vi "Write Data Type.vi"(8 "error in (no error)":errorcluster, 10 "Data Type":T1, 11 "OnChange_Boolean in":refnum<class "OnChangeNotifier_I8.lvclass">) -> (0 "error out":errorcluster, 3 "OnChange_Boolean out":refnum<class "OnChangeNotifier_I8.lvclass">)   [LabVIEW 2021, in "OnChangeNotifier_I8.lvclass"]
uses:
  OnChangeNotifier_I8.lvclass
  Support/Class Type.ctl
  OnChangeNotifier_I8.lvclass/OnChangeNotifier_I8.ctl
  <vilib>/TSA/Abstract Data Classes/Abs_Types/I8 Integer/Abs_I8 Integer.lvclass
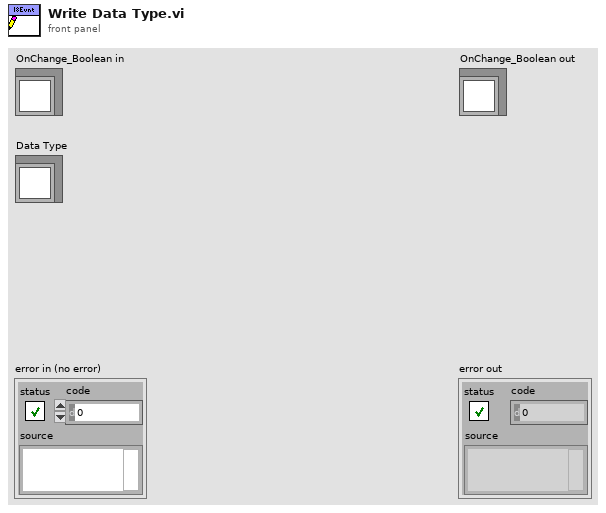
[diagram p1: front panel]
types:
  T1 = typedef "OnChangeNotifier_I8.lvclass/Class Type.ctl" = refnum<class "Abs_I8 Integer.lvclass">
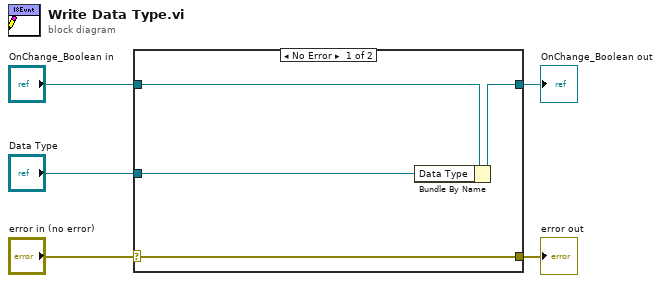
[diagram p0: block diagram]
diagram:
  n1 = case shown="No Error" "error in (no error)" {
    selector: "error in (no error)" -> [w9 w10]
    tunnel: [w9 w10] -> w4
    tunnel: [w7 w11] -> w2
    tunnel: "OnChange_Boolean in" -> [w8 w11]
    tunnel: "Data Type" -> [w6 _]
    frame No Error {
      n2 = Bundle By Name(cluster=w8, "Data Type"=w6) -> (w7:refnum<class "OnChangeNotifier_I8.lvclass">)
    }
    frame Error {
    }
  }
  "error out" <- w4
  "OnChange_Boolean out" <- w2
